vi "Send Tag SetRequest_ByRef.vi"(4 "Timeout (-1)":i32=-1, 6 "Synchronous (F)":bool, 8 "error in (no error)":errorcluster, 9 "Value":variant, 10 "Tag Ref in":refnum<data-value>) -> (0 "error out":errorcluster, 1 "timed out?":bool, 2 "Tag Ref out":refnum<data-value>)   [LabVIEW 2020, in "Tag Engine.lvlib"]
doc: "_SubVI_"
uses:
  Tag Engine.lvlib
  Tag/Tag.lvclass
  Tag/Tag.lvclass/Tag.ctl
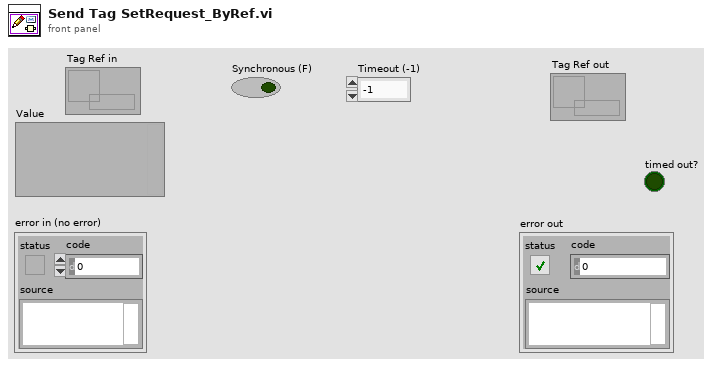
[diagram p1: front panel]
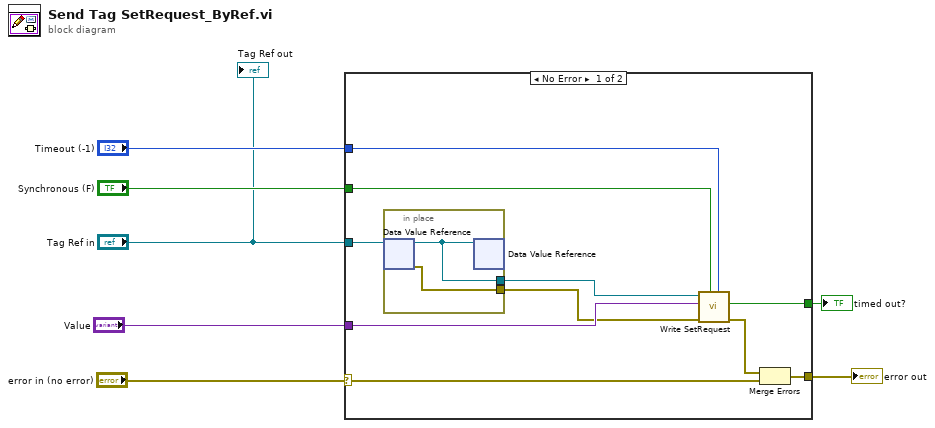
[diagram p0: block diagram]
diagram:
  n1 = case shown="No Error" "error in (no error)" {
    selector: "error in (no error)" -> [w16 w20]
    tunnel: "Tag Ref in" -> [w17 _]
    tunnel: [w15 w20] -> w7
    tunnel: "Value" -> [w14 _]
    tunnel: "Synchronous (F)" -> [w13 _]
    tunnel: "Timeout (-1)" -> [w12 _]
    tunnel: [w9 _] -> w4
    frame No Error {
      n2 = in-place {
        in-place-border: [w19] -> w11
        in-place-border: [w18] -> w8
        n3 = in-place-dvr #1(w17) -> (w18:refnum<class "Tag.lvclass">, w19:errorcluster)
        n4 = in-place-dvr #1(w18) -> ()  [unwired: 2 out]
      }
      n5 = call "Write SetRequest.vi"("Timeout (-1)"=w12, "Synchronous (F)"=w13, "error in (no error)"=w11, "Value"=w14, "Tag in"=w8) -> ("error out"=w10:errorcluster, "timed out?"=w9:bool)  [unwired: 4 in, 1 out]
      n6 = Merge Errors(w10, w16) -> (w15:errorcluster)
    }
    frame Error {
    }
  }
  "error out" <- w7
  "timed out?" <- w4
  "Tag Ref out" <- "Tag Ref in"
